vi "Untitled 7 (SubVI).vi"(11 "Boolean in":refnum<vi>) -> ()   [LabVIEW 2021]
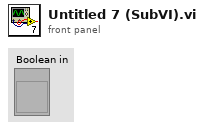
[diagram p1: front panel]
types:
  T1 = enum8{"Enabled", "Disabled", "Disabled and Grayed Out"}
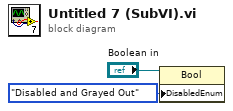
[diagram p0: block diagram]
diagram:
  n1 = property on="Property Node" class="Bool"(reference="Boolean in", "DisabledEnum"=T1."Disabled and Grayed Out" ("Disabled")) -> ()  [unwired: 1 in, 2 out]
